vi "wait.vi"(0 "HGF_Occurrence":refnum<class "HGF_Occurrence.lvclass">, 3 "msTimeout (-1)":i32=-1, 5 "error in (no error)":errorcluster, 9 "ignore previous (F)":bool) -> (14 "dup HGF_Occurrence":refnum<class "HGF_Occurrence.lvclass">, 16 "Object":refnum<class>, 17 "timed out":bool, 19 "error out":errorcluster)   [LabVIEW 2014, in "HGF_BaseClasses.lvlib" / "HGF_Occurrence.lvclass"]
doc: "Use this VI to wait on events.\n\n<b>Hint:</b> This is a shared reentrant VI."
uses:
  HGF_Occurrence.lvclass
  HGF_Event/HGF_Event.lvclass
  HGF_Timing/HGF_Timing.lvclass
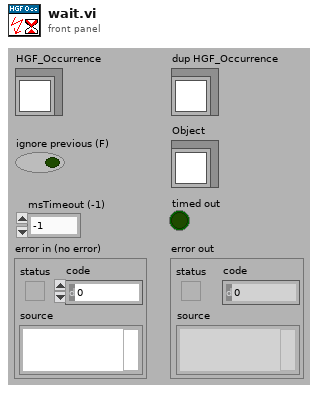
[diagram p1: front panel]
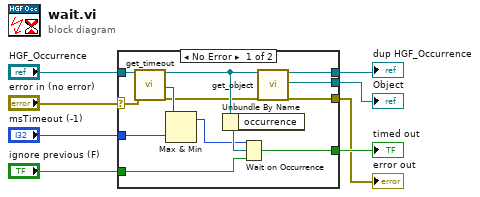
[diagram p0: block diagram]
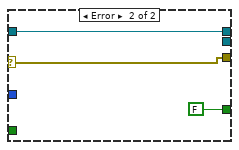
[diagram p2: hidden frame]
diagram:
  n1 = case shown="No Error" "error in (no error)" {
    selector: "error in (no error)" -> [w20 w23]
    tunnel: "HGF_Occurrence" -> [w21 w24]
    tunnel: [w13 w24] -> w4
    tunnel: "msTimeout (-1)" -> [w18 _]
    tunnel: "ignore previous (F)" -> [w15 _]
    tunnel: [w12 _] -> w3
    tunnel: [w10 FALSE ("timed out")] -> w2
    tunnel: [w9 w23] -> w1
    frame No Error {
      n2 = call "get_timeout.vi"("HGF_Event.lvclass in"=w21, "error in (no error)"=w20) -> ("HGF_Event.lvclass out"=w14:refnum<class "HGF_Occurrence.lvclass">, "timeout"=w19:i32, "error out"=w11:errorcluster)  [unwired: 15 out]
      n3 = Max & Min(x=w19, y=w18) -> (max(x,y)=w16:i32)  [unwired: 1 out]
      n4 = Unbundle By Name(w14) -> ("occurrence"=w17:refnum<k4>)
      n5 = Wait on Occurrence(1:w15, 2:w17, 3:w16) -> (0:w10:bool)
      n6 = call "get_object.vi"("HGF_Timing.lvclass"=w14, "error in (no error)"=w11) -> ("dup HGF_Timing"=w13:refnum<class "HGF_Occurrence.lvclass">, "object"=w12:refnum<class>, "error out"=w9:errorcluster)  [unwired: 15 out]
    }
    frame Error {
    }
  }
  "error out" <- w1
  "dup HGF_Occurrence" <- w4
  "timed out" <- w2
  "Object" <- w3
